vi "Update UI Display.vi"(8 "error in (no error)":errorcluster, 10 "Update for Display":string, 11 "References":T1) -> (0 "error out":errorcluster)   [LabVIEW 2021, in "Build Script Common.lvlib"]
uses:
  Build Script Common.lvlib
  Typedef/References.ctl
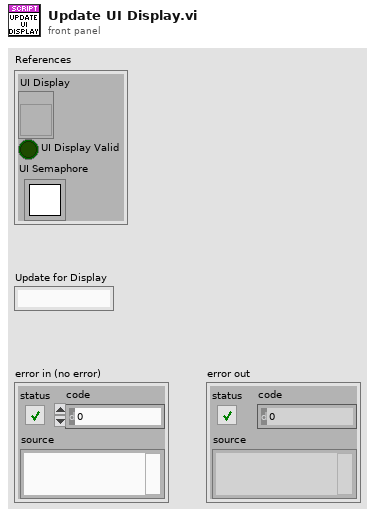
[diagram p1: front panel]
types:
  T1 = typedef "Build Script Common.lvlib/References.ctl" = cluster{"UI Display":refnum<vi>, "UI Display Valid":bool, "UI Semaphore":T2}
  T2 = typedef "Semaphore RefNum" = refnum<k1>
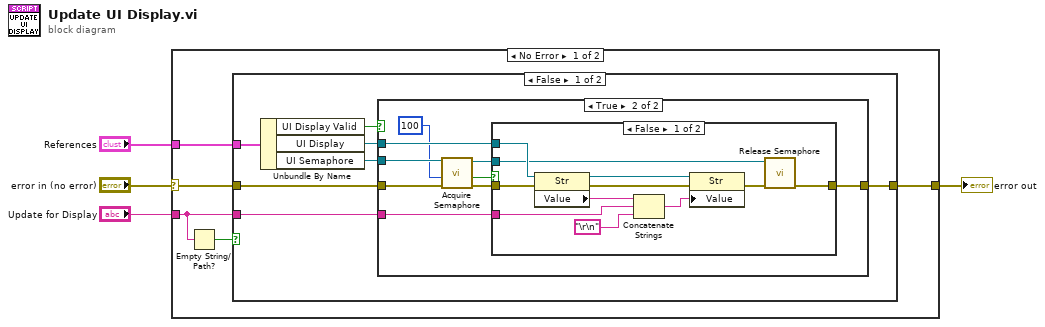
[diagram p0: block diagram]
diagram:
  n1 = case shown="No Error" "error in (no error)" {
    selector: "error in (no error)" -> [w9 w40]
    tunnel: "Update for Display" -> [w6 _]
    tunnel: [w8 w40] -> w2
    tunnel: "References" -> [w7 _]
    frame No Error {
      n2 = Empty String/Path?(string/path=w6) -> (empty?=w5:bool)
      n3 = case shown="False" w5 {
        tunnel: w6 -> [w16 _]
        tunnel: w9 -> [w15 w39]
        tunnel: [w14 w39] -> w8
        tunnel: w7 -> [w13 _]
        frame False {
          n4 = Unbundle By Name(w13) -> ("UI Display Valid"=w12:bool, "UI Display"=w11:refnum<vi>, "UI Semaphore"=w10:T2)
          n5 = case shown="True" w12 {
            tunnel: w16 -> [_ w26]
            tunnel: w15 -> [w17 w23]
            tunnel: [w17 w25] -> w14
            tunnel: w11 -> [_ w24]
            tunnel: w10 -> [_ w21]
            frame False {
            }
            frame True {
              n6 = call <vilib>:"Acquire Semaphore.vi"("error in (no error)"=w23, "ms timeout (-1)"=100, "semaphore"=w21) -> ("error out"=w22:errorcluster, "timed out"=w19:bool, "semaphore out"=w18:T2)  [unwired: 2 in]
              n7 = case shown="False" w19 {
                tunnel: w26 -> [w28 _]
                tunnel: [w30 w38] -> w25
                tunnel: w24 -> [w33 _]
                tunnel: w22 -> [w32 w38]
                tunnel: w18 -> [w29 _]
                frame False {
                  n8 = property class="Str"(reference=w33, error in=w32) -> (reference out=w35:refnum<vi>, error out=w34:errorcluster, "Value"=w37:string)
                  n9 = Concatenate Strings(w37, w28, "\r\n") -> (w36:string)
                  n10 = property class="Str"(reference=w35, error in=w34, "Value"=w36) -> (error out=w31:errorcluster)  [unwired: 1 out]
                  n11 = call <vilib>:"Release Semaphore.vi"("error in (no error)"=w31, "semaphore"=w29) -> ("error out"=w30:errorcluster)  [unwired: 4 in, 1 out]
                }
                frame True {
                }
              }
            }
          }
        }
        frame True {
        }
      }
    }
    frame Error {
    }
  }
  "error out" <- w2
